vi "FGV_Boolean.vi"(8 "error in":errorcluster, 9 "点亮":bool, 10 "状态":enum16{"Init", "Read", "Write"}(ring)) -> (0 "error out":errorcluster, 2 "点亮":bool)   [LabVIEW 2020]
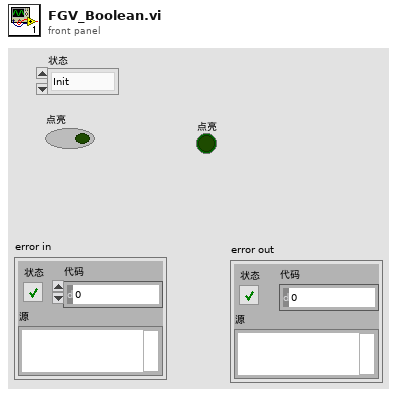
[diagram p1: front panel]
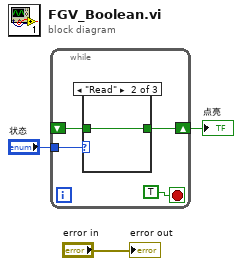
[diagram p0: block diagram]
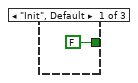
[diagram p2: hidden frame]
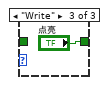
[diagram p3: hidden frame]
diagram:
  n1 = while {
    tunnel: "状态" -> [w6]
    shift-right: [w5] -> w1
    shift-left: _ -> [w4]
    stop <- TRUE stop-if-true
    n2 = case shown="\"Read\"" w6 {
      tunnel: [FALSE w9 "点亮"] -> w5
      tunnel: w4 -> [_ w9 _]
      frame "Init", Default {
      }
      frame "Read" {
      }
      frame "Write" {
      }
    }
  }
  "点亮" <- w1
  "error out" <- "error in"
